vi "Move Elves.vi"(0 "Elves in":set{T1}(c389), 1 "Elves' Movement Proposals":map{T1, T1}(c390)) -> (2 "Elves out":set{T1}(c389))   [LabVIEW 2020, in "AoC 2022.lvlib"]
uses:
  AoC 2022.lvlib
  Day 15 - Beacon Exclusion Zone/private/Location.ctl
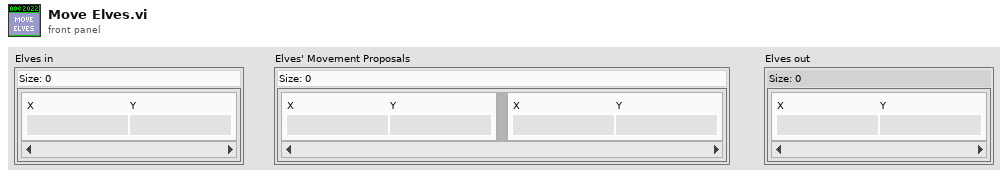
[diagram p1: front panel]
types:
  T1 = typedef "AoC 2022.lvlib/Location.ctl" = cluster{"X":i32, "Y":i32}
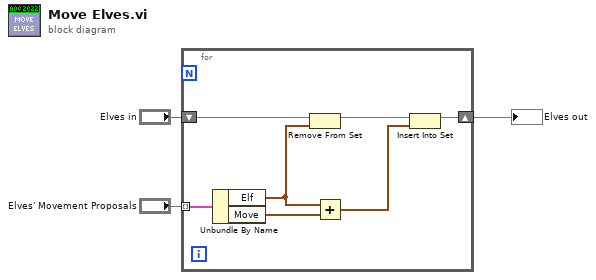
[diagram p0: block diagram]
diagram:
  n1 = for {
    tunnel: "Elves' Movement Proposals" -> [w10] mode=indexing
    shift-right: [w4] -> w1
    shift-left: "Elves in" -> [w8]
    n2 = Unbundle By Name(w10) -> ("Elf"=w7:T1, "Move"=w9:T1)
    n3 = Remove From Set(10:w7, 11:w8) -> (3:w6:set{T1})  [unwired: 1 out]
    n4 = Add(x=w7, y=w9) -> (x+y=w5:T1)
    n5 = Insert Into Set(10:w5, 11:w6) -> (3:w4:set{T1})  [unwired: 1 out]
  }
  "Elves out" <- w1
